vi "DS18b20_ReadID.vi"(8 "error in (no error)":errorcluster) -> (0 "error out":errorcluster, 3 "standard output":string)   [LabVIEW 2014, in "QwaveSys RPi Training Library.lvlib"]
uses:
  <vilib>/Q-Wave Systems/QwaveSys RPi Package 2.0/Addons/QwaveSys RPi Training Library.lvlib
panel:
  out "standard error":string
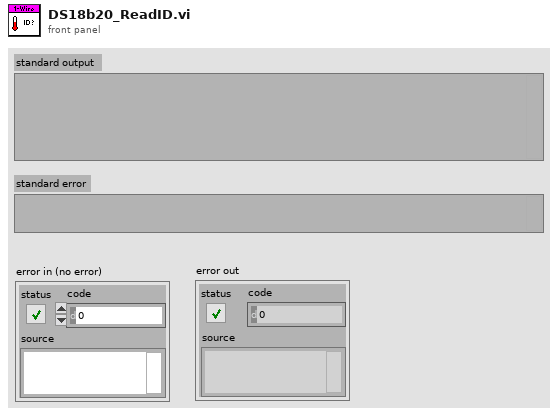
[diagram p1: front panel]
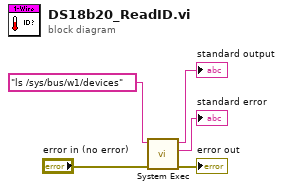
[diagram p0: block diagram]
diagram:
  n1 = call <vilib>:"System Exec.vi"("error in (no error)"="error in (no error)", "command line"="ls /sys/bus/w1/devices") -> ("error out"=→"error out":errorcluster, "standard error"=→"standard error":string, "standard output"=→"standard output":string)  [unwired: 6 in, 1 out]
